vi "Main.vi"() -> ()   [LabVIEW 2013]
doc: "This Continuous Measurement sample project is based on the Queued Message Handler template.\n\nThe Event Handling Loop generates messages based on user interface actions.\n\nThe Message Handling Loop processes messages generated by the Event Handling Loop, or by other messages. There are also Acquisition and Logging message handling loop subVIs, and a chart updating loop."
uses:
  Settings/Settings.ctl
  Acquisition/Hardware Configuration.ctl
  Acquisition/Signal Type.ctl
  Logging/Logging Configuration.ctl
  controls/UI Data.ctl
  controls/UI State.ctl
  <vilib>/Utility/error.llb/DialogType.ctl
  support/Message Queue/Enqueue Message (Single).vi
  <vilib>/Utility/error.llb/Error Cluster From Error Code.vi
  <vilib>/ErrorRing/Error Ring.xnode
  Acquisition/Acquisition.lvlib
  Logging/Logging.lvlib
  Settings/Settings.lvlib
  support/User Event - Stop/User Event - Stop.lvlib
  support/Message Queue/Message Queue.lvlib
  support/Message Queue/Message Cluster.ctl
  support/Message Queue/Enqueue Message (MultiLine String w Array).vi
panel:
  out "Data":waveform(dbl)[](graph)
  in  "Settings":bool
  in  "Start":bool
  in  "Stop":bool
  out "Status":string
  in  "Exit":bool
  # "Continuous Measurement Data Logger"
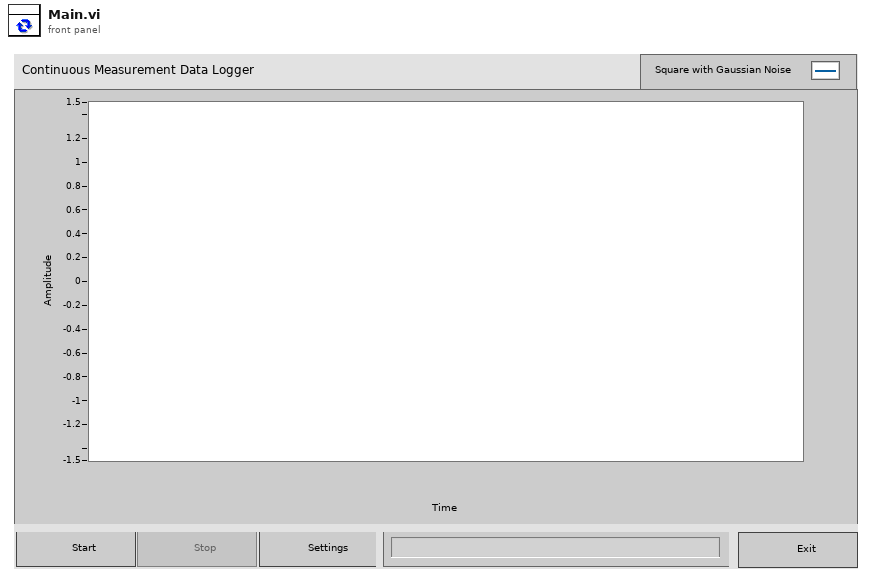
[diagram p1: front panel]
types:
  T1 = cluster{"Macro:Initialize":string, "Macro:Exit":string, "Core":cluster{"Current VI Reference":refnum<vi>, "Close Panel on Exit?":bool}}
  T2 = typedef "UI State.ctl" = enum16{"Idle", "Acquiring and Logging", "Waiting for Exit", "Waiting for Exit (Acq Stopped)", "Waiting for Exit (Log Stopped)", "Waiting for Stop", "Waiting for Stop (Acq Stopped)", "Waiting for Stop (Log Stopped)"}
  T3 = typedef "UI Data.ctl" = cluster{"Start Ref":refnum<vi>, "Stop Ref":refnum<vi>, "Settings Ref":refnum<vi>, "Exit Ref":refnum<vi>, "Status Ref":refnum<vi>, "Data Ref":refnum<vi>}
  T4 = typedef "Settings.lvlib/Settings.ctl" = cluster{"Hardware Configuration":T5, "Logging Configuration":T7}
  T5 = typedef "Acquisition.lvlib/Hardware Configuration.ctl" = cluster{"HW Refnum <Replace Me>":string, "Signal Type <Replace Me>":T6}
  T6 = typedef "Acquisition.lvlib/Signal Type.ctl" = enum16{"Sine Wave", "Square with Noise"}
  T7 = typedef "Logging.lvlib/Logging Configuration.ctl" = cluster{"Log File Base Path":path, "TDMS File Reference":refnum<k34>}
  T8 = typedef "Message Queue.lvlib/All Message Queues.ctl" = cluster{"UI":refnum<queue>, "Acquisition":refnum<queue>, "Logging":refnum<queue>}
  T9 = enum32{"invalid app kind", "Development System", "Run Time System", "Student Edition", "Embedded LabVIEW", "Evaluation", "Custom"}
  T10 = enum32{"Invalid", "Standard", "Closed", "Hidden", "Minimized", "Maximized"}
  T11 = typedef "DialogType.ctl" = u16
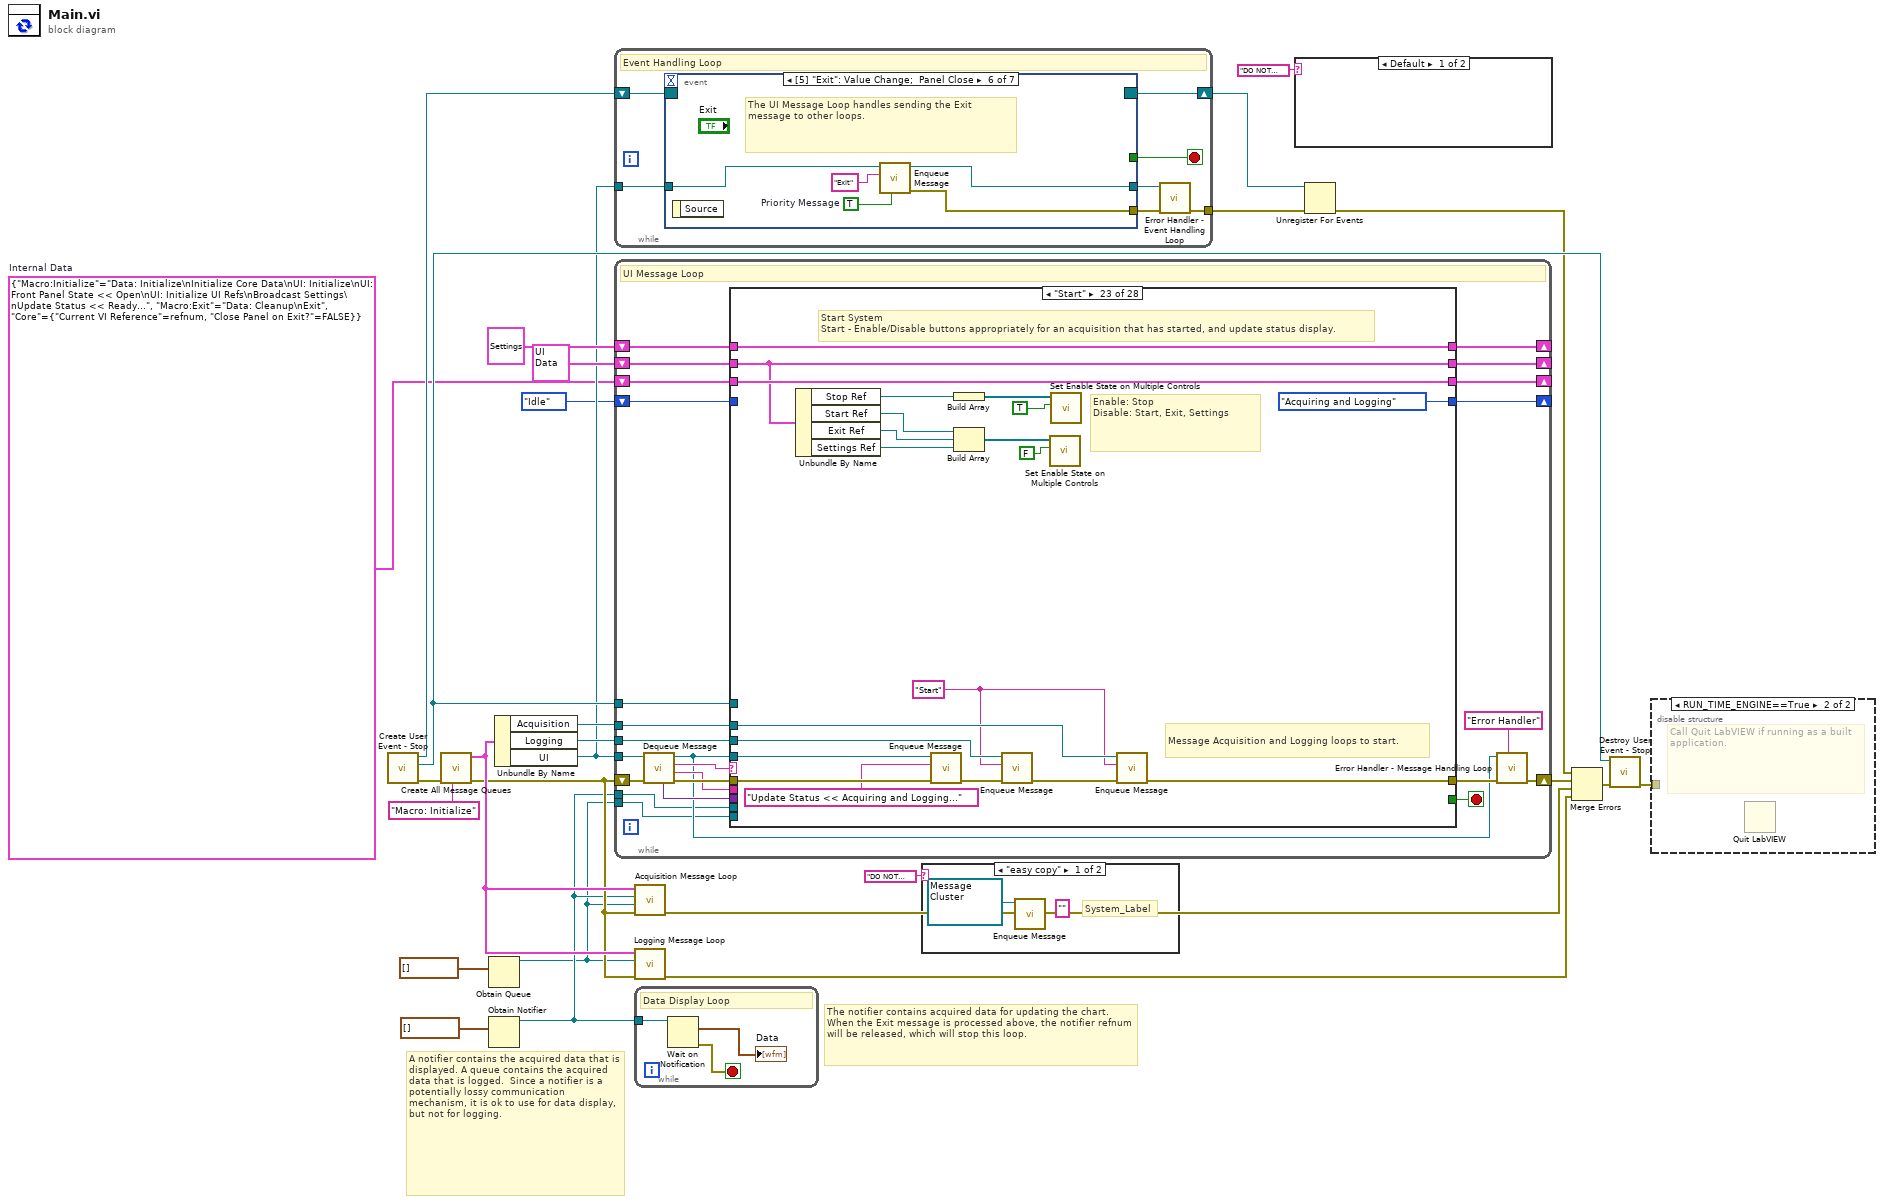
[diagram p0: block diagram]
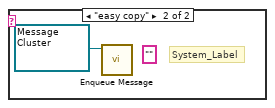
[diagram p2: hidden frame]
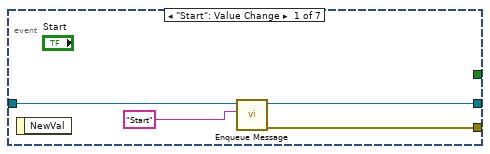
[diagram p5: hidden frame]
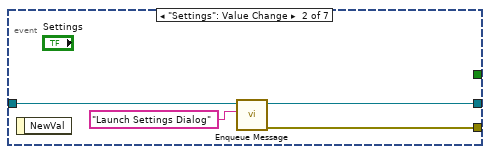
[diagram p6: hidden frame]
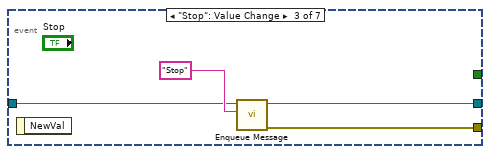
[diagram p7: hidden frame]
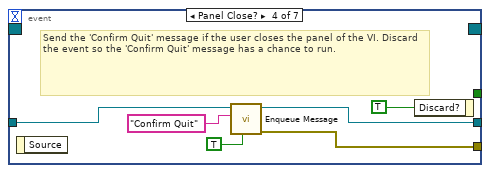
[diagram p8: hidden frame]
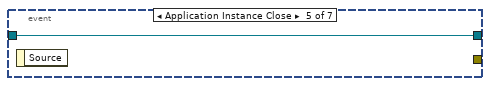
[diagram p9: hidden frame]
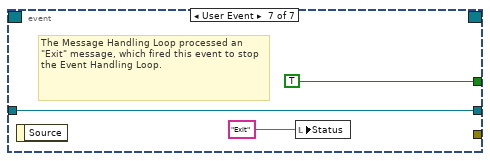
[diagram p10: hidden frame]
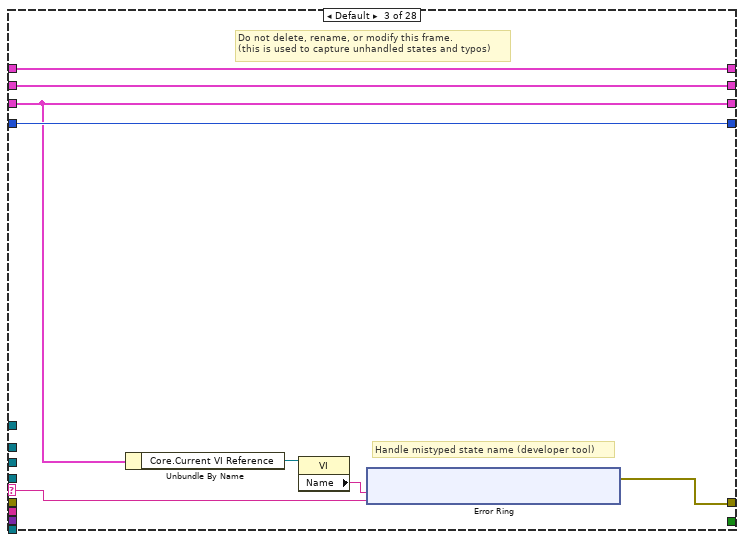
[diagram p13: hidden frame]
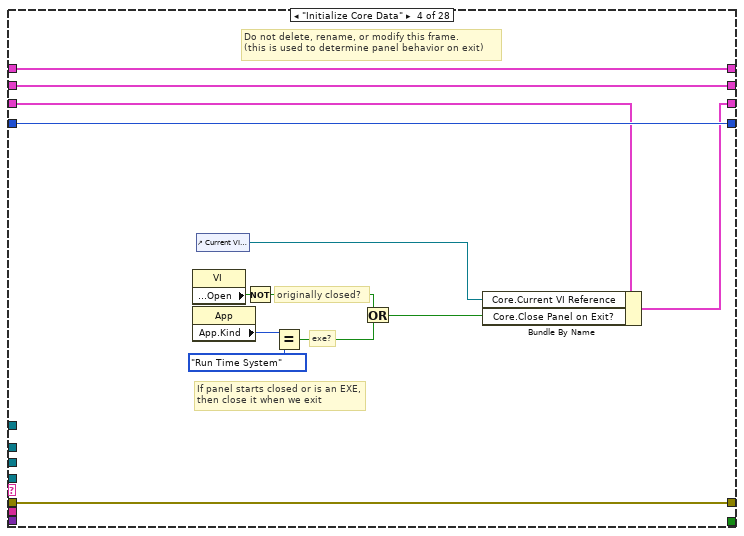
[diagram p14: hidden frame]
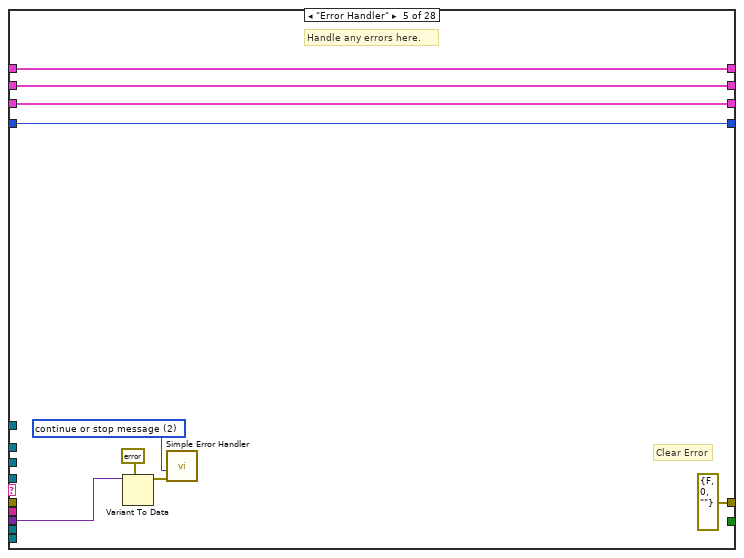
[diagram p15: hidden frame]
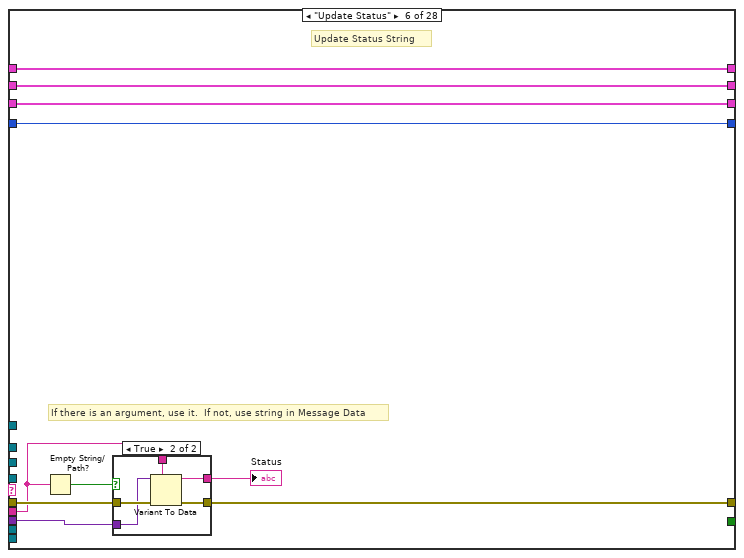
[diagram p16: hidden frame]
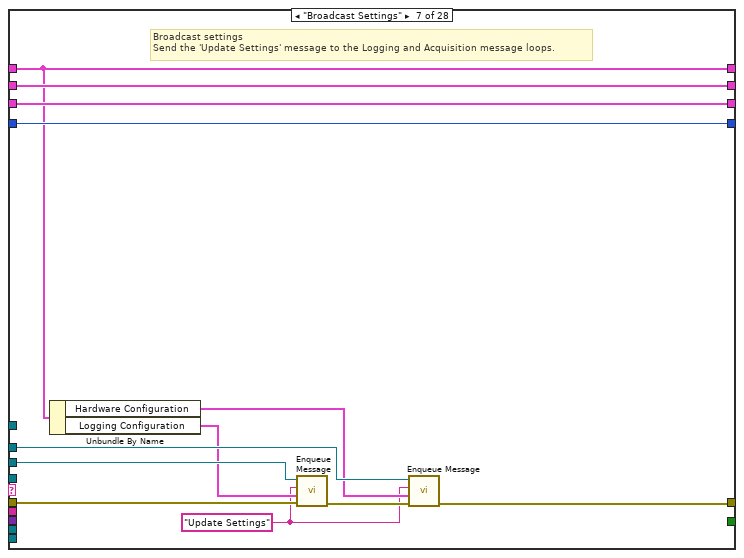
[diagram p18: hidden frame]
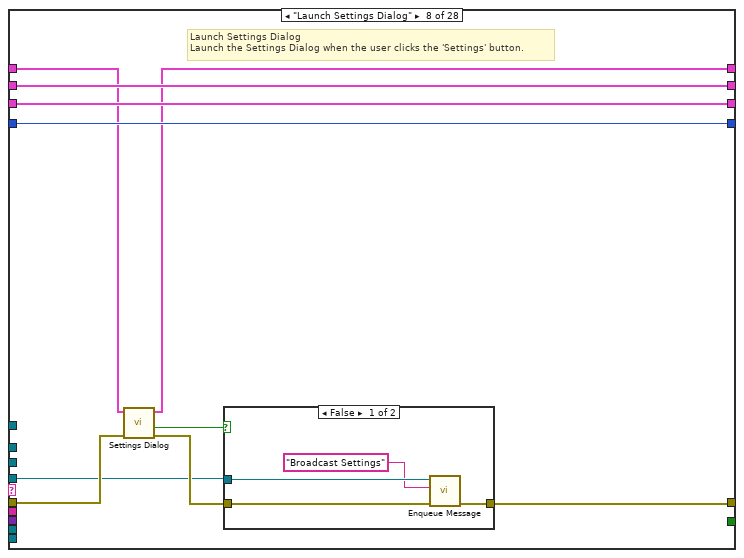
[diagram p19: hidden frame]
diagram:
  w4 = T1 {"Macro:Initialize"="Data: Initialize\nInitialize Core Data\nUI: Initialize\nUI: Front Panel State << Open\nUI: Initialize UI Refs\nBroadcast Settings\nUpdate Status << Ready...", "Macro:Exit"="Data: Cleanup\nExit", "Core"={"Current VI Reference"=refnum, "Close Panel on Exit?"=FALSE}}  # Internal Data
  # "A notifier contains the acquired data that is displayed. A queue contains the acquired data that is logged.  Since a notifier is a potentially lossy communication mechanism, it is ok to use for data display, but not for logging."
  # "The notifier contains acquired data for updating the chart. When the Exit message is processed above, the notifier refnum will be released, which will stop this loop."
  n1 = call "Create User Event - Stop.vi"() -> ("error out"=w22:errorcluster, "User Event - Stop"=w24:refnum<user-event>, "Stop Event Registration Refnum"=w25:refnum<event-registration>)  [unwired: 9 in]
  n2 = call "Create All Message Queues.vi"("Message"="Macro: Initialize", "error in (no error)"=w22) -> ("error out"=w19:errorcluster, "Message Queues out"=w21:T8)  [unwired: 8 in]
  n3 = Obtain Queue(element data type=waveform(dbl)[] []) -> (queue out=w8:refnum<queue>)  [unwired: 4 in, 2 out]
  n4 = Obtain Notifier(notification data type=waveform(dbl)[] []) -> (notifier out=w10:refnum<notifier>)  [unwired: 3 in, 2 out]
  n5 = Unbundle By Name(w21) -> ("Acquisition"=w14:refnum<queue>, "Logging"=w13:refnum<queue>, "UI"=w12:refnum<queue>)
  n6 = while {
    tunnel: w12 -> [w33]
    tunnel: [w30] -> w26
    shift-right: [w32] -> w16
    shift-left: w25 -> [w34]
    stop <- w31 stop-if-true
    # "Event Handling Loop"
    n7 = event shown="[5] \"Exit\": Value Change;  Panel Close" {
      selector: w34 -> [_ _ _ _ _ _ _]
      dyn-events: [_ _ _ _ _ _ _] -> w32
      timeout: _ -> [_ _ _ _ _ _ _]
      tunnel: [_ _ _ _ _ _ TRUE ("Discard?")] -> w31
      tunnel: w33 -> [w38 w40 w45 w50 w53 w55 w59]
      tunnel: [w36 w42 w44 w48 _ w58 _] -> w29
      tunnel: [w35 w39 w43 w49 w53 w54 w59] -> w28
      event "Start": Value Change {
        n8 = event-data() -> ()  [unwired: 1 in, 1 out]
        n9 = call-poly "Enqueue Message.vi"("Message"="Start", "Message Queue"=w38) -> ("error out"=w36:errorcluster, "dup Message Queue"=w35:refnum<queue>)  [unwired: 8 in]
      }
      event "Settings": Value Change {
        n10 = event-data() -> ()  [unwired: 1 in, 1 out]
        n11 = call-poly "Enqueue Message.vi"("Message"="Launch Settings Dialog", "Message Queue"=w40) -> ("error out"=w42:errorcluster, "dup Message Queue"=w39:refnum<queue>)  [unwired: 8 in]
      }
      event "Stop": Value Change {
        n12 = event-data() -> ()  [unwired: 1 in, 1 out]
        n13 = call-poly "Enqueue Message.vi"("Message"="Stop", "Message Queue"=w45) -> ("error out"=w44:errorcluster, "dup Message Queue"=w43:refnum<queue>)  [unwired: 8 in]
      }
      event Panel Close? {
        # "Send the 'Confirm Quit' message if the user closes the panel of the VI. Discard the event so the 'Confirm Quit' message has a chance to run."
        n14 = event-data() -> ()  [unwired: 1 in, 1 out]
        n15 = call-poly "Enqueue Message.vi"("Priority Message? (F)"=TRUE, "Message"="Confirm Quit", "Message Queue"=w50) -> ("error out"=w48:errorcluster, "dup Message Queue"=w49:refnum<queue>)  [unwired: 7 in]
        n16 = event-data("Discard?"=TRUE) -> ()  [unwired: 1 in, 1 out]
      }
      event Application Instance Close {
        n17 = event-data() -> ()  [unwired: 1 in, 1 out]
      }
      event "Exit": Value Change; Panel Close {
        w56 = TRUE  # Priority Message
        # "The UI Message Loop handles sending the Exit message to other loops."
        n18 = event-data() -> ()  [unwired: 1 in, 1 out]
        n19 = call-poly "Enqueue Message.vi"("Priority Message? (F)"=w56, "Message"="Exit", "Message Queue"=w55) -> ("error out"=w58:errorcluster, "dup Message Queue"=w54:refnum<queue>)  [unwired: 7 in]
      }
      event User Event {
        # "The Message Handling Loop processed an \"Exit\" message, which fired this event to stop the Event Handling Loop."
        n20 = event-data() -> ()  [unwired: 1 in, 1 out]
        n21 = local write "Status"("Exit" ("Exit String")) -> ()
      }
    }
    n22 = call "Error Handler - Event Handling Loop.vi"("error in (no error)"=w29, "Message Queue"=w28) -> ("dup error in"=w30:errorcluster)  [unwired: 8 in, 1 out]
  }
  n23 = while {
    tunnel: w12 -> [w84]
    tunnel: w24 -> [w80]
    shift-right: [w83] -> w27
    shift-left: w19 -> [w85]
    shift-right: [w71] -> _
    shift-left: T4 {"Hardware Configuration"={"HW Refnum <Replace Me>"="", "Signal Type <Replace Me>"=enum."Sine Wave"}, "Logging Configuration"={"Log File Base Path"=path "", "TDMS File Reference"=refnum}} ("Settings") -> [w73]
    shift-right: [w70] -> _
    shift-left: T3 {"Start Ref"=refnum, "Stop Ref"=refnum, "Settings Ref"=refnum, "Exit Ref"=refnum, "Status Ref"=refnum, "Data Ref"=refnum} ("Measurement UI Controls") -> [w72]
    tunnel: w14 -> [w79]
    tunnel: w13 -> [w78]
    tunnel: w10 -> [w63]
    tunnel: w8 -> [w62]
    shift-right: [w77] -> _
    shift-left: UI_State."Idle" ("UI State") -> [w76]
    shift-right: [w66] -> _
    shift-left: w4 -> [w67]
    stop <- w75 stop-if-true
    # "UI Message Loop"
    n24 = call "Dequeue Message.vi"("error in (no error)"=w85, "Message Queue"=w84) -> ("error out"=w82:errorcluster, "Argument"=w69:string, "Message"=w81:string, "dup Message Queue"=w65:refnum<queue>, "Message Data"=w68:variant)  [unwired: 5 in]
    n25 = case shown="\"Start\"" w81 {
      selector: w81 -> [_ _ w97 _ _ _ _ _ _ _ _ _ _ _ _ _ _ _ _ _ w330 _ _ _ _ _ _ _]
      tunnel: w72 -> [w89 w93 w102 w116 w133 w142 w162 w172 w185 w222 w227 w236 w239 w246 w251 w263 w276 w287 w317 w326 w345 w351 w372 w392 w402 w428 w451 w456]
      tunnel: w69 -> [_ _ _ _ _ w135 _ _ _ _ _ _ _ _ _ _ w277 w288 _ _ _ _ _ _ _ _ _ _]
      tunnel: w73 -> [w88 w94 w103 w114 w131 w143 w155 w169 w179 w224 w228 w234 w240 w247 w253 w273 w280 w290 w318 w327 w343 w352 w374 w394 w404 w430 w452 w457]
      tunnel: [w90 w95 w96 w124 errorcluster {"status"=FALSE, "code"=0, "source"=""} ("error out") w137 w151 w163 w178 w214 w229 w232 w241 w248 w252 w272 w278 w291 w319 w322 w332 w353 w355 w375 w399 w423 w453 w458] -> w74
      tunnel: w82 -> [w90 w95 _ w124 _ w139 w159 w167 w182 w212 w229 w233 w242 w248 w252 w272 w279 w292 w319 w324 w342 w353 w362 w377 w400 w424 w453 w458]
      tunnel: [w89 w93 w102 w116 w133 w142 w162 w172 w185 w222 w227 w236 w239 w246 w251 w254 w276 w287 w317 w326 w345 w351 w372 w392 w402 w428 w451 w456] -> w70
      tunnel: [_ _ _ _ _ _ _ _ _ TRUE _ _ _ _ _ _ _ _ _ _ _ _ _ _ _ _ _ _] -> w75
      tunnel: [w88 w94 w103 w114 w131 w143 w155 w168 w179 w224 w228 w231 w240 w247 w253 w273 w280 w290 w318 w327 w343 w352 w374 w394 w404 w430 w452 w457] -> w71
      tunnel: w80 -> [_ _ _ _ _ _ _ _ _ w213 _ _ _ _ _ _ _ _ _ _ _ _ _ _ _ _ _ _]
      tunnel: w79 -> [_ _ _ _ _ _ w156 _ _ w211 _ _ _ _ _ _ _ _ _ _ w328 _ w357 w382 _ _ _ _]
      tunnel: w78 -> [_ _ _ _ _ _ w158 _ _ w210 _ _ _ _ _ _ _ _ _ _ w329 _ w359 w383 _ _ _ _]
      tunnel: [w87 w92 w101 w115 w132 w141 w161 w171 w180 UI_State."Idle" ("UI State") w226 w235 w238 w245 w250 w271 w275 w286 w316 w325 w344 w350 UI_State."Acquiring and Logging" ("UI State") w378 w398 w426 w450 w455] -> w77
      tunnel: w76 -> [w87 w92 w101 w115 w132 w141 w161 w171 w181 _ w226 w235 w238 w245 w250 w271 w275 w286 w316 w325 w344 w350 _ w379 w397 w427 w450 w455]
      tunnel: w68 -> [_ _ _ _ w127 w138 _ _ _ _ _ _ _ _ _ _ _ _ _ _ _ _ _ _ _ _ _ _]
      tunnel: w67 -> [w86 w91 w99 w113 w130 w140 w160 w170 w184 w221 w225 w230 w237 w244 w249 w270 w274 w285 w315 w320 w336 w349 w373 w393 w403 w429 w449 w454]
      tunnel: [w86 w91 w99 w112 w130 w140 w160 w170 w184 w221 w225 w230 w237 w244 w249 w270 w274 w285 w315 w320 w336 w349 w373 w393 w403 w429 w449 w454] -> w66
      tunnel: w65 -> [_ _ _ _ _ _ _ w164 w183 w209 _ _ _ _ _ _ _ _ _ w323 w341 _ w361 _ w401 w425 _ _]
      tunnel: w63 -> [_ _ _ _ _ _ _ _ _ w208 _ _ _ _ _ _ _ _ _ _ _ _ _ _ _ _ _ _]
      tunnel: w62 -> [_ _ _ _ _ _ _ _ _ w207 _ _ _ _ _ _ _ _ _ _ _ _ _ _ _ _ _ _]
      frame "", "Idle" {
        # "Executes when the state queue is empty\nAlso commented out messages"
      }
      frame "---------- Core ----------" {
        # "Do not put any code in this frame.\n(it is a separator no-op)"
      }
      frame Default {
        # "Handle mistyped state name (developer tool)"
        # "Do not delete, rename, or modify this frame.\n(this is used to capture unhandled states and typos)"
        n26 = Unbundle By Name(w99) -> ("Core.Current VI Reference"=w98:refnum<vi>)
        n27 = property class="VI"(reference=w98) -> ("Name"=w100:string)  [unwired: 1 in, 2 out]
        n28 = xnode "Error Ring"("parameter 0"=w100, "parameter 1"=w97) -> ("error out"=w96:errorcluster)
      }
      frame "Initialize Core Data" {
        # "Do not delete, rename, or modify this frame.\n(this is used to determine panel behavior on exit)"
        # "originally closed?"
        # "exe?"
        # "If panel starts closed or is an EXE, then close it when we exit"
        n29 = property class="VI"() -> ("Front Panel.Open"=w123:bool)  [unwired: 2 in, 2 out]
        n30 = property class="App"() -> ("App.Kind"=w122:T9)  [unwired: 2 in, 2 out]
        n31 = control-ref of="Current VI Reference"() -> (w117:refnum<vi>)
        n32 = Not(x=w123) -> (.not. x?=w120:bool)
        n33 = Equal?(x=w122, y=T9."Run Time System" ("Application:Kind")) -> (x = y?=w119:bool)
        n34 = Or(x=w120, y=w119) -> (x .or. y?=w118:bool)
        n35 = Bundle By Name(cluster=w113, "Core.Current VI Reference"=w117, "Core.Close Panel on Exit?"=w118) -> (w112:T1)
      }
      frame "Error Handler" {
        w126 = T11 2 items=["no dialog", "OK message", "continue or stop message", "OK message + warnings", "continue/stop + warnings"] ("type of dialog (OK msg:1)")
        # "Clear Error"
        # "Handle any errors here."
        n36 = Variant To Data(type=errorcluster {"status"=FALSE, "code"=0, "source"=""} ("error constant"), Variant=w127) -> (data=w129:errorcluster)  [unwired: 1 in, 1 out]
        n37 = call <vilib>:"Simple Error Handler.vi"("type of dialog (OK msg:1)"=w126, "error in (no error)"=w129) -> ()  [unwired: 3 in, 5 out]
      }
      frame "Update Status" {
        # "If there is an argument, use it.  If not, use string in Message Data"
        # "Update Status String"
        n38 = Empty String/Path?(string/path=w135) -> (empty?=w136:bool)
        n39 = case shown="True" w136 {
          tunnel: w139 -> [w144 w150]
          tunnel: w138 -> [_ w149]
          tunnel: w135 -> [w145 w148]
          tunnel: [w144 w147] -> w137
          tunnel: [w145 w146] -> w134
          frame False {
          }
          frame True {
            n40 = Variant To Data(error in=w150, type=w148, Variant=w149) -> (data=w146:string, error out=w147:errorcluster)
          }
        }
        "Status" <- w134
      }
      frame "Broadcast Settings" {
        w152 = "Update Settings" ("Message")
        # "Broadcast settings\nSend the 'Update Settings' message to the Logging and Acquisition message loops."
        n41 = Unbundle By Name(w155) -> ("Hardware Configuration"=w153:T5, "Logging Configuration"=w154:T7)
        n42 = call-poly "Enqueue Message.vi"("error in (no error)"=w159, "Message Data"=w154, "Message"=w152, "Message Queue"=w158) -> ("error out"=w157:errorcluster)  [unwired: 6 in, 1 out]
        n43 = call-poly "Enqueue Message.vi"("error in (no error)"=w157, "Message Data"=w153, "Message"=w152, "Message Queue"=w156) -> ("error out"=w151:errorcluster)  [unwired: 6 in, 1 out]
      }
      frame "Launch Settings Dialog" {
        # "Launch Settings Dialog\nLaunch the Settings Dialog when the user clicks the 'Settings' button."
        n44 = call "Settings Dialog.vi"("error in (no error)"=w167, "Settings in"=w169) -> ("error out"=w165:errorcluster, "Cancelled?"=w166:bool, "Settings out"=w168:T4)  [unwired: 6 in, 1 out]
        n45 = case shown="False" w166 {
          tunnel: w164 -> [w176 _]
          tunnel: w165 -> [w175 w177]
          tunnel: [w174 w177] -> w163
          frame False {
            n46 = call-poly "Enqueue Message.vi"("error in (no error)"=w175, "Message"="Broadcast Settings", "Message Queue"=w176) -> ("error out"=w174:errorcluster)  [unwired: 7 in, 1 out]
          }
          frame True {
          }
        }
      }
      frame "Confirm Quit" {
        # "Confirm Quit\nMessage that can confirm whether or not the user wants to exit the application."
        n47 = case shown="\"Acquiring and Logging\"" w181 {
          tunnel: w183 -> [w191 w195]
          tunnel: w182 -> [w190 w194]
          tunnel: [w189 w193] -> w178
          tunnel: [UI_State."Idle" ("UI State") w192] -> w180
          frame Default {
            # "If 'Confirm Quit' comes in while the system is idle, there is no need for a confirmation message."
            n48 = call-poly "Enqueue Message.vi"("Priority Message? (F)"=TRUE, "error in (no error)"=w190, "Message"="Exit", "Message Queue"=w191) -> ("error out"=w189:errorcluster)  [unwired: 6 in, 1 out]
          }
          frame "Acquiring and Logging" {
            n49 = Two Button Dialog(message="Are you sure you want to quit while the acquisition is running?" ("Confirm Quit Message"), 1:"No" ("No"), 2:"Yes" ("Yes")) -> (T button?=w196:bool)
            n50 = case shown="True" w196 {
              tunnel: w195 -> [_ w205]
              tunnel: w194 -> [w201 w206]
              tunnel: [w201 w204] -> w193
              tunnel: [UI_State."Acquiring and Logging" ("UI State") UI_State."Waiting for Exit" ("UI State")] -> w192
              frame False {
                # "User did not want to quit."
              }
              frame True {
                n51 = call-poly "Enqueue Message.vi"("error in (no error)"=w206, "Message"="Stop", "Message Queue"=w205) -> ("error out"=w204:errorcluster)  [unwired: 7 in, 1 out]
              }
            }
          }
        }
      }
      frame "Exit" {
        w219 = "Exit" ("Message")
        # "Don't check the error outs. The acquisition and logging queues may have already been released."
        # "Close references owned by the Main VI."
        # "Stop the VI"
        # "Exit\nFire the User Event to stop the Event Handling Loop.  Also send Exit messages to the Acquisition and Logging loops."
        n52 = Release Queue(queue=w209, error in (no error)=w212) -> (error out=w218:errorcluster)  [unwired: 1 in, 2 out]
        n53 = call "Fire User Event - Stop.vi"("User Event - Stop"=w213) -> ("error out"=w220:errorcluster)  [unwired: 10 in]
        n54 = Release Notifier(notifier=w208, error in (no error)=w218) -> (error out=w217:errorcluster)  [unwired: 1 in, 2 out]
        n55 = Release Queue(queue=w207, error in (no error)=w217) -> (error out=w216:errorcluster)  [unwired: 1 in, 2 out]
        n56 = call-poly "Enqueue Message.vi"("Message"=w219, "Message Queue"=w211) -> ()  [unwired: 8 in, 2 out]
        n57 = call-poly "Enqueue Message.vi"("Message"=w219, "Message Queue"=w210) -> ()  [unwired: 8 in, 2 out]
        n58 = Merge Errors(w220, w216) -> (w214:errorcluster)
      }
      frame "---------- Data ----------" {
        # "Do not put any code in this frame.\n(It is a separator no-op. You can make a copy of this frame to create a new Data frame)"
      }
      frame "Data: Initialize" {
        # "nothing right now"
        # "Initialize the shift-register data, here.\n(data names are defined by what you wire into the bundle function)"
        n59 = call "Load Settings from XML.vi"("error in (no error)"=w233, "Settings in"=w234) -> ("error out"=w232:errorcluster, "Settings out"=w231:T4)  [unwired: 8 in]
      }
      frame "Data: Cleanup" {
        # "Cleanup any data and references, here.\n(this is called automatically, by the Macro: Exit)"
        n60 = Unbundle By Name(w237) -> ("Core.Current VI Reference"=w243:refnum<vi>)
        n61 = Close Reference(reference=w243, error in (no error)=w242) -> (error out=w241:errorcluster)
      }
      frame "---------- UI ----------" {
        # "Do not put any code in this frame.\n(It is a separator no-op. You can make a copy of this frame to create a new UI frame)"
      }
      frame "UI: Initialize" {
        # "Initialize the User Interface, here.\n(this is called automatically, by the Macro: Init)"
      }
      frame "UI: Initialize UI Refs" {
        # "Enable: Start, Exit, Settings\nDisable: Stop"
        # "Package and Init UI Refs as Required"
        n62 = control-ref of="Data"() -> (w264:refnum<vi>)
        n63 = control-ref of="Start"() -> (w269:refnum<vi>)
        n64 = control-ref of="Stop"() -> (w267:refnum<vi>)
        n65 = control-ref of="Settings"() -> (w268:refnum<vi>)
        n66 = control-ref of="Exit"() -> (w266:refnum<vi>)
        n67 = control-ref of="Status"() -> (w265:refnum<vi>)
        n68 = Bundle By Name(cluster=w263, "Start Ref"=w269, "Stop Ref"=w267, "Settings Ref"=w268, "Exit Ref"=w266, "Status Ref"=w265, "Data Ref"=w264) -> (w254:T3)
        n69 = Unbundle By Name(w254) -> ("Stop Ref"=w262:refnum<vi>, "Start Ref"=w259:refnum<vi>, "Exit Ref"=w258:refnum<vi>, "Settings Ref"=w257:refnum<vi>)
        n70 = Build Array(w262) -> (w261:refnum<vi>[])
        n71 = Build Array(w259, w258, w257) -> (w256:refnum<vi>[])
        n72 = call "Set Enable State on Multiple Controls.vi"("Enable?"=TRUE, "Controls"=w256) -> ()  [unwired: 10 in]
        n73 = call "Set Enable State on Multiple Controls.vi"("Enable?"=FALSE, "Controls"=w261) -> ()  [unwired: 10 in]
      }
      frame "UI: Cursor Set" {
        # "Argument"
        # "Set and Unset Cursor Busy.\n(Usage: \"UI: Cursor Set >> Busy|Idle\")"
        n74 = case shown="\"Idle\", Default" w277 {
          tunnel: w279 -> [w282 w284]
          tunnel: [w281 w283] -> w278
          frame "Idle", Default {
            n75 = call <vilib>:"Unset Busy.vi"("error in (no error)"=w282) -> ("error out"=w281:errorcluster)  [unwired: 10 in]
          }
          frame "Busy" {
            n76 = call <vilib>:"Set Busy.vi"("error in (no error)"=w284) -> ("error out"=w283:errorcluster)  [unwired: 9 in, 1 out]
          }
        }
      }
      frame "UI: Front Panel State" {
        # "Argument"
        # "Set Front Panel Open or Closed\n(Usage: \"UI: Front Panel State >> Open|Close\")"
        n77 = Unbundle By Name(w285) -> ("Core.Current VI Reference"=w289:refnum<vi>)
        n78 = case shown="\"Open\", Default" w288 {
          tunnel: w292 -> [w296 w309]
          tunnel: [w298 w310] -> w291
          tunnel: w289 -> [w297 w307]
          frame "Open", Default {
            n79 = property class="VI"(reference=w297, error in=w296) -> (reference out=w294:refnum<vi>, error out=w295:errorcluster, "Front Panel.Open"=w293:bool)
            n80 = case shown="True" w293 {
              tunnel: [w301 w304] -> w298
              tunnel: w295 -> [w300 w304]
              tunnel: w294 -> [w299 _]
              frame False {
                n81 = invoke class="VI" method="FP.Open"(reference=w299, error in=w300, "Activate"=TRUE, "State"=T10."Standard") -> (error out=w301:errorcluster)  [unwired: 1 in, 4 out]
              }
              frame True {
              }
            }
          }
          frame "Close" {
            n82 = property class="VI"(reference=w307, error in=w309) -> (reference out=w306:refnum<vi>, error out=w308:errorcluster, "Front Panel.Open"=w305:bool)
            n83 = case shown="True" w305 {
              tunnel: [w311 w314] -> w310
              tunnel: w308 -> [w311 w313]
              tunnel: w306 -> [_ w312]
              frame False {
              }
              frame True {
                n84 = invoke class="VI" method="FP.Close"(reference=w312, error in=w313) -> (error out=w314:errorcluster)  [unwired: 1 in, 2 out]
              }
            }
          }
        }
      }
      frame "---------- Macro ----------" {
        # "Do not put any code in this frame.\n(It is a separator no-op. You can make a copy of this frame to create a new Macro frame)"
      }
      frame "Macro: Initialize" {
        # "Initialization Macro\n(This is called once, when the VI starts)"
        n85 = Unbundle By Name(w320) -> ("Macro:Initialize"=w321:string)
        n86 = call-poly "Enqueue Message.vi"("error in (no error)"=w324, "Message"=w321, "Message Queue"=w323) -> ("error out"=w322:errorcluster)  [unwired: 7 in, 1 out]
      }
      frame "Macro: Exit" {
        w331 = FALSE ("Priority Message? (F)")
        # "Exit Macro\n(This is called once, when the VI exits)"
        n87 = Unbundle By Name(w336) -> ("Core.Close Panel on Exit?"=w348:bool)
        n88 = Unbundle By Name(w336) -> ("Macro:Exit"=w335:string)
        n89 = Select(t="UI: Front Panel State >> Close", s=w348, f="") -> (s? t:f=w340:string)
        n90 = call-poly "Enqueue Message.vi"("Priority Message? (F)"=TRUE, "error in (no error)"=w342, "Message"=w340, "Message Queue"=w341) -> ("error out"=w337:errorcluster, "dup Message Queue"=w338:refnum<queue>)  [unwired: 6 in]
        n91 = call-poly "Enqueue Message.vi"("Priority Message? (F)"=w331, "error in (no error)"=w337, "Message"=w335, "Message Queue"=w338) -> ("error out"=w334:errorcluster)  [unwired: 6 in, 1 out]
        n92 = call-poly "Enqueue Message.vi"("Priority Message? (F)"=w331, "error in (no error)"=w334, "Message"=w330, "Message Queue"=w329) -> ("error out"=w333:errorcluster)  [unwired: 6 in, 1 out]
        n93 = call-poly "Enqueue Message.vi"("Priority Message? (F)"=w331, "error in (no error)"=w333, "Message"=w330, "Message Queue"=w328) -> ("error out"=w332:errorcluster)  [unwired: 6 in, 1 out]
      }
      frame "---------- System ----------" {
        # "Template Separator\n(You can make a copy of, or modify, this frame)"
      }
      frame "Start" {
        w354 = "Start" ("Message")
        # "Message Acquisition and Logging loops to start."
        # "Enable: Stop\nDisable: Start, Exit, Settings"
        # "Start System\nStart - Enable/Disable buttons appropriately for an acquisition that has started, and update status display."
        n94 = Unbundle By Name(w372) -> ("Stop Ref"=w371:refnum<vi>, "Start Ref"=w368:refnum<vi>, "Exit Ref"=w367:refnum<vi>, "Settings Ref"=w366:refnum<vi>)
        n95 = call-poly "Enqueue Message.vi"("error in (no error)"=w362, "Message"="Update Status << Acquiring and Logging...", "Message Queue"=w361) -> ("error out"=w358:errorcluster)  [unwired: 7 in, 1 out]
        n96 = Build Array(w371) -> (w370:refnum<vi>[])
        n97 = Build Array(w368, w367, w366) -> (w365:refnum<vi>[])
        n98 = call-poly "Enqueue Message.vi"("error in (no error)"=w358, "Message"=w354, "Message Queue"=w359) -> ("error out"=w356:errorcluster)  [unwired: 7 in, 1 out]
        n99 = call "Set Enable State on Multiple Controls.vi"("Enable?"=FALSE, "Controls"=w365) -> ()  [unwired: 10 in]
        n100 = call "Set Enable State on Multiple Controls.vi"("Enable?"=TRUE, "Controls"=w370) -> ()  [unwired: 10 in]
        n101 = call-poly "Enqueue Message.vi"("error in (no error)"=w356, "Message"=w354, "Message Queue"=w357) -> ("error out"=w355:errorcluster)  [unwired: 7 in, 1 out]
      }
      frame "Stop" {
        w380 = "Stop" ("Message")
        # "Message Acquisition and Logging loops to stop"
        # "Enable: Start, Exit, Settings\nDisable: Stop"
        # "Stop System\nEnable/Disable buttons appropriately for an acquisition that has stopped, and update status display."
        n102 = Unbundle By Name(w392) -> ("Stop Ref"=w391:refnum<vi>, "Start Ref"=w388:refnum<vi>, "Exit Ref"=w387:refnum<vi>, "Settings Ref"=w386:refnum<vi>)
        n103 = Build Array(w391) -> (w390:refnum<vi>[])
        n104 = Build Array(w388, w387, w386) -> (w385:refnum<vi>[])
        n105 = call-poly "Enqueue Message.vi"("error in (no error)"=w377, "Message"=w380, "Message Queue"=w383) -> ("error out"=w381:errorcluster)  [unwired: 7 in, 1 out]
        n106 = call "Set Enable State on Multiple Controls.vi"("Enable?"=TRUE, "Controls"=w385) -> ()  [unwired: 10 in]
        n107 = call "Set Enable State on Multiple Controls.vi"("Enable?"=FALSE, "Controls"=w390) -> ()  [unwired: 10 in]
        n108 = call-poly "Enqueue Message.vi"("error in (no error)"=w381, "Message"=w380, "Message Queue"=w382) -> ("error out"=w376:errorcluster)  [unwired: 7 in, 1 out]
        n109 = Merge Errors(w376) -> (w375:errorcluster)
        n110 = case shown="Default" w379 {
          selector: w379 -> [w395 _]
          tunnel: [w395 UI_State."Waiting for Stop" ("UI State")] -> w378
          frame "Waiting for Exit" {
          }
          frame Default {
          }
        }
      }
      frame "Acquisition Stopped" {
        # "Logic for determining what action to take when the acquisition has stopped."
        n111 = case shown="\"Waiting for Stop (Log Stopped)\"" w397 {
          selector: w397 -> [w406 _ _ _ _]
          tunnel: w400 -> [w405 w408 w410 w416 w422]
          tunnel: w401 -> [_ _ _ w414 w419]
          tunnel: [w406 UI_State."Waiting for Exit (Acq Stopped)" ("UI State") UI_State."Waiting for Stop (Acq Stopped)" ("UI State") UI_State."Idle" ("UI State") UI_State."Idle" ("UI State")] -> w398
          tunnel: [w405 w408 w410 w415 w420] -> w399
          frame Default {
          }
          frame "Waiting for Exit", "Waiting for Exit (Acq Stopped)" {
          }
          frame "Waiting for Stop", "Waiting for Stop (Acq Stopped)" {
          }
          frame "Waiting for Exit (Log Stopped)" {
            # "If we are waiting to exit, and the logging has already stopped, then the \"Acquisition Stopped\" message indicates that it is time to exit."
            n112 = call-poly "Enqueue Message.vi"("Priority Message? (F)"=TRUE, "error in (no error)"=w416, "Message"="Exit", "Message Queue"=w414) -> ("error out"=w415:errorcluster)  [unwired: 6 in, 1 out]
          }
          frame "Waiting for Stop (Log Stopped)" {
            # "If we are waiting to stop, and the logging has already stopped, then the \"Acquisition Stopped\" message indicates that it is time to stop."
            n113 = call-poly "Enqueue Message.vi"("error in (no error)"=w422, "Message Data"="Ready..." ("Ready..."), "Message"="Update Status", "Message Queue"=w419) -> ("error out"=w420:errorcluster)  [unwired: 6 in, 1 out]
          }
        }
      }
      frame "Logging Stopped" {
        # "Logic for determining what action to take when the logging has stopped."
        n114 = case shown="\"Waiting for Stop (Acq Stopped)\"" w427 {
          selector: w427 -> [w432 _ _ _ _]
          tunnel: w424 -> [w431 w434 w436 w442 w445]
          tunnel: w425 -> [_ _ _ w440 w444]
          tunnel: [w432 UI_State."Waiting for Exit (Log Stopped)" ("UI State") UI_State."Waiting for Stop (Log Stopped)" ("UI State") UI_State."Idle" ("UI State") UI_State."Idle" ("UI State")] -> w426
          tunnel: [w431 w434 w436 w441 w443] -> w423
          frame Default {
          }
          frame "Waiting for Exit", "Waiting for Exit (Log Stopped)" {
          }
          frame "Waiting for Stop", "Waiting for Stop (Log Stopped)" {
          }
          frame "Waiting for Exit (Acq Stopped)" {
            # "If we are waiting to exit, and the acquisition has already stopped, then the \"Logging Stopped\" message indicates that it is time to exit."
            n115 = call-poly "Enqueue Message.vi"("Priority Message? (F)"=TRUE, "error in (no error)"=w442, "Message"="Exit", "Message Queue"=w440) -> ("error out"=w441:errorcluster)  [unwired: 6 in, 1 out]
          }
          frame "Waiting for Stop (Acq Stopped)" {
            # "If we are waiting to stop, and the acquisition has already stopped, then the \"Logging Stopped\" message indicates that it is time to stop."
            n116 = call-poly "Enqueue Message.vi"("error in (no error)"=w445, "Message Data"="Ready..." ("Ready..."), "Message"="Update Status", "Message Queue"=w444) -> ("error out"=w443:errorcluster)  [unwired: 6 in, 1 out]
          }
        }
      }
      frame "---------- New Category ----------" {
        # "Template Separator\n(You can make a copy of, or modify, this frame)"
      }
      frame "New Category: 1" {
        # "Your code here.\n(You can make a copy of, or modify, this frame)"
      }
    }
    n117 = call "Error Handler - Message Handling Loop.vi"("Error Handler Message"="Error Handler" ("Message"), "error in (no error)"=w74, "Message Queue"=w65) -> ("dup error in"=w83:errorcluster)  [unwired: 7 in, 1 out]
  }
  n118 = call "Acquisition Message Loop.vi"("error in (no error)"=w19, "Data Queue"=w8, "Data Notifier"=w10, "Message Queues"=w21) -> ("error out"=w23:errorcluster)  [unwired: 7 in]
  n119 = call "Logging Message Loop.vi"("error in (no error)"=w19, "Data Queue"=w8, "Message Queues"=w21) -> ("error out"=w20:errorcluster)  [unwired: 8 in]
  n120 = while "Data Display Loop" {
    tunnel: w10 -> [w461]
    stop <- w459 stop-if-true
    # "Data Display Loop"
    n121 = Wait on Notification(notifier=w461) -> (notification=→"Data":waveform(dbl)[], error out=w459:errorcluster)  [unwired: 3 in, 2 out]
  }
  n122 = case shown="\"easy copy\"" "DO NOT RUN!!" {
    frame "easy copy" {
      (unwired) "" ("Message")
      # "System_Label"
      n123 = call-poly "Enqueue Message.vi"("Message Queue"=refnum<queue> refnum) -> ()  [unwired: 9 in, 2 out]
    }
    frame Default {
    }
  }
  n124 = case shown="Default" "DO NOT RUN!!" {
    frame Default {
    }
    frame "easy copy" {
      (unwired) "" ("Message")
      # "System_Label"
      n125 = call-poly "Enqueue Message.vi"("Message Queue"=refnum<queue> refnum) -> ()  [unwired: 9 in, 2 out]
    }
  }
  n126 = Unregister For Events(event registration refnum=w16, error in=w26) -> (error out=w17:errorcluster)
  n127 = Merge Errors(w17, w27, w23, w20) -> (w5:errorcluster)
  n128 = call "Destroy User Event - Stop.vi"("error in (no error)"=w5, "User Event - Stop"=w24) -> ("error out"=w7:errorcluster)  [unwired: 9 in]
  n129 = disable-structure shown="RUN_TIME_ENGINE==True" {
    disable-tunnel: w7 -> [_ _]
    frame condition #0 (active) {
    }
    frame condition #1 {
      # "Call Quit LabVIEW if running as a built application."
      n130 = Quit LabVIEW() -> ()  [unwired: 1 in]
    }
  }
